vi "niRFUtil WFM Apply Logrithmic Gain (real array).vi"(1 "Gain, dB":sgl=1.0 format="%.2f", 3 "Signal In, dBm":T1 min=0 max=127 format="%.2f") -> (0 "Signal Out, dBm":T1 min=0 max=127 format="%.2f")   [LabVIEW 2015, in "niRFUtil.lvlib"]
doc: "(c) Copyright 2006, National Instruments, Inc. This VI may not be duplicated, sold, or distributed without written consent from National Instruments."
uses:
  niRFUtil.lvlib
  Includes/niRFUtil INC Real Array.ctl
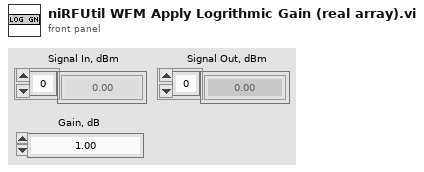
[diagram p1: front panel]
types:
  T1 = typedef "niRFUtil.lvlib/niRFUtil INC Real Array.ctl" = sgl[]
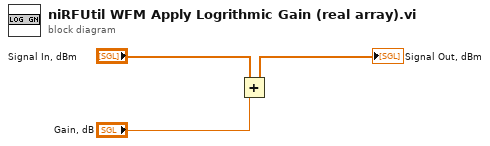
[diagram p0: block diagram]
diagram:
  n1 = Add(x="Signal In, dBm", y="Gain, dB") -> (x+y=→"Signal Out, dBm":T1)
